vi "Auto Zoom.vi"(8 "error in":errorcluster, 9 "Stop":dbl, 10 "Start":dbl, 11 "Instrument Handle In":i32) -> (0 "error out":errorcluster, 3 "Instrument Handle Out":i32)   [LabVIEW 8.6, in "ZTScopeM.lvlib"]
doc: "Configure the auto download buffer zoom level. A start and stop that are equal to the capture time (0 to sweep time) will cause a single waveform to be available in the auto download buffer. A different start and stop time will provide a secondary \"zoomed\" waveform within the selected times."
uses:
  ZTScopeM.lvlib
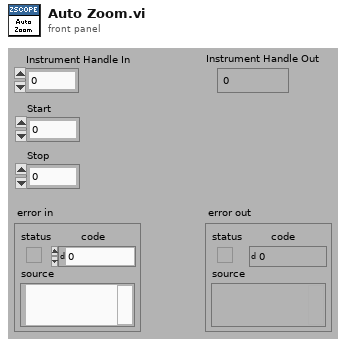
[diagram p1: front panel]
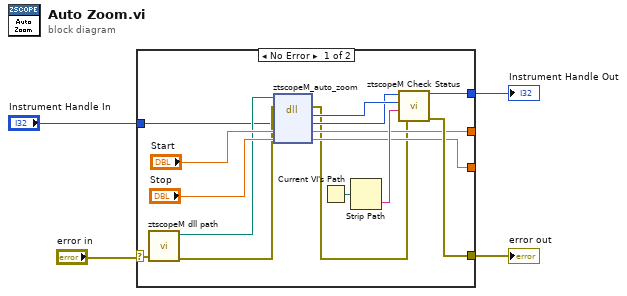
[diagram p0: block diagram]
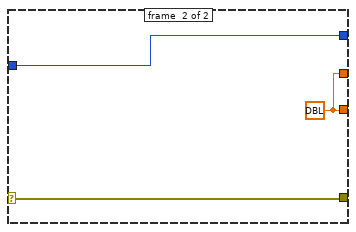
[diagram p2: hidden frame]
diagram:
  n1 = case shown="No Error" "error in" {
    selector: "error in" -> [w9 w22]
    tunnel: [w14 w22] -> w3
    tunnel: [w15 w20] -> w2
    tunnel: [w12 w21] -> _
    tunnel: [w10 w21] -> _
    tunnel: "Instrument Handle In" -> [w5 w20]
    frame #0 {
      n2 = call "ztscopeM dll path.vi"("error in (no error)"=w9) -> ("error out"=w7:errorcluster, "<instrument>.dll path"=w8:path)  [unwired: 9 in]
      n3 = dll-call lib="C:/Program Files (x86)/National Instruments/LabVIEW 2013/instr.lib/ztscopem/ztscopeM.dll" fn="ztscopeM_auto_zoom"(path in=w8, error in=w7, "instrumentHandle"=w5, "Start"="Start", "Stop"="Stop") -> (error out=w6:errorcluster, w19:i32, "instrumentHandle"=w18:i32, "Start"=w10:dbl, "Stop"=w12:dbl)  [unwired: 1 in, 1 out]
      n4 = Current VI's Path() -> (path=w17:path)
      n5 = Strip Path(path=w17) -> (name=w16:string)  [unwired: 1 out]
      n6 = call "ztscopeM Check Status.vi"("error in"=w6, "name of VI"=w16, "status (return code)"=w19, "instrument handle in"=w18) -> ("error out"=w14:errorcluster, "instrument handle out"=w15:i32)  [unwired: 2 out]
    }
    frame #1 {
      w21 = dbl ? ("Stop")
    }
  }
  "Instrument Handle Out" <- w2
  "error out" <- w3
